vi "Get Current Day as Timestamp.vi"() -> (1 "Day as String (YYYY-MM-DD)":string, 2 "Time Stamp":timestamp format="%<%x %.3X>T")   [LabVIEW 2020, in "Time Management.lvlib"]
doc: "Returns the current day as a Timestamp. The timestamp will be rounded to the nearest factor of a day in seconds (86400). Since the beginning time in LabVIEW is January 1, 1904 12:00 am universal time, the specific time referenced will be related to your timezone referenced to univerasl time.\n\n08/2025, Erich Schlieper"
uses:
  Time Management.lvlib
  <vilib>/Utility/miscctls.llb/LVDateTimeRec.ctl
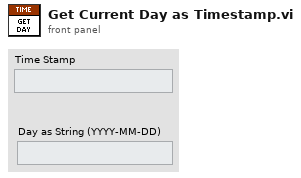
[diagram p1: front panel]
types:
  T1 = typedef "LVDateTimeRec.ctl" = cluster{"fractional second":dbl, "second":i32, "minute":i32, "hour":i32, "day of month":i32, "month":i32, "year":i32, "day of week":i32, "day of year":i32, "DST":i32}
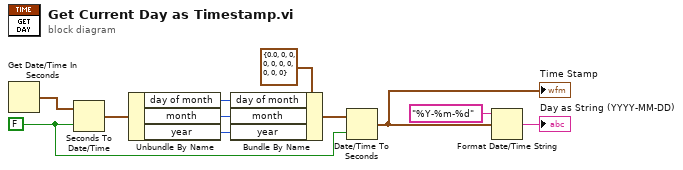
[diagram p0: block diagram]
diagram:
  w2 = FALSE ("to UTC (F)")
  n1 = Get Date/Time In Seconds() -> (seconds since 1Jan1904=w9:timestamp)
  n2 = Seconds To Date/Time(time stamp (now)=w9, to UTC (F)=w2) -> (date time rec=w7:T1)
  n3 = Unbundle By Name(w7) -> ("day of month"=w6:i32, "month"=w5:i32, "year"=w4:i32)
  n4 = Bundle By Name(cluster=T1 {"fractional second"=0.0, "second"=0, "minute"=0, "hour"=0, "day of month"=0, "month"=0, "year"=0, "day of week"=0, "day of year"=0, "DST"=0} ("date time rec"), "day of month"=w6, "month"=w5, "year"=w4) -> (w3:T1)
  n5 = Date/Time To Seconds(1:w2, 2:w3) -> (0:w1:timestamp)
  "Time Stamp" <- w1
  n6 = Format Date/Time String(time format string (%c)="%Y-%m-%d", seconds (now)=w1) -> (date/time string=→"Day as String (YYYY-MM-DD)":string)  [unwired: 1 in]
